vi "Create G-CLI Script VIPCApply.vi"(8 "error in (no error)":errorcluster, 10 "VIPC File Path":path, 11 "PostBuildSupport in":refnum<class "PostBuildSupport.lvclass">) -> (0 "error out":errorcluster, 2 "command":string, 3 "PostBuildSupport out":refnum<class "PostBuildSupport.lvclass">)   [LabVIEW 2019, in "PostBuildSupport.lvclass"]
uses:
  PostBuildSupport.lvclass
  PostBuildSupport.lvclass/PostBuildSupport.ctl
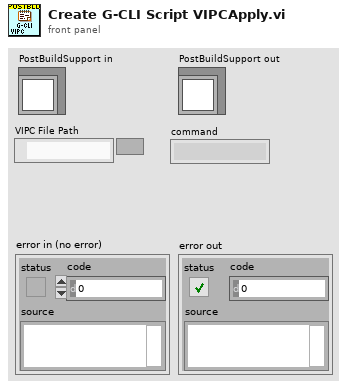
[diagram p1: front panel]
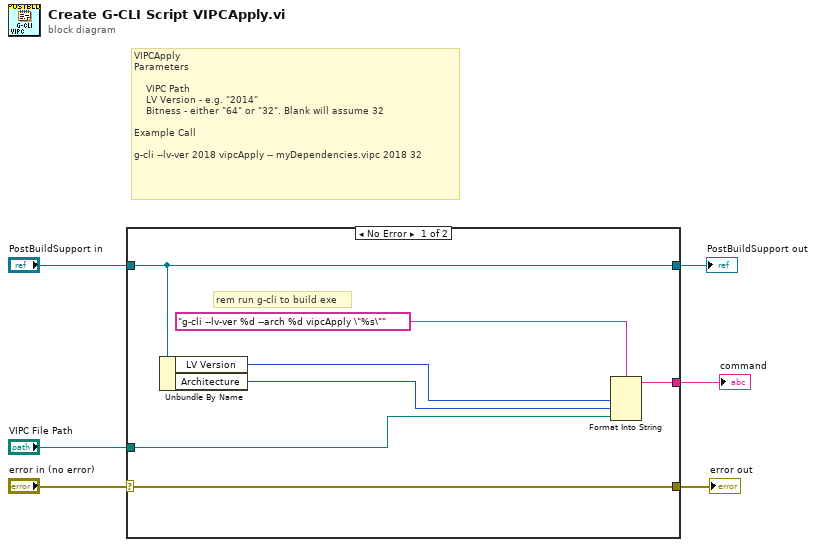
[diagram p0: block diagram]
diagram:
  # "VIPCApply\nParameters\n\n    VIPC Path\n    LV Version - e.g. \"2014\"\n    Bitness - either \"64\" or \"32\". Blank will assume 32\n\nExample Call\n\ng-cli --lv-ver 2018 vipcApply -- myDependencies.vipc 2018 32"
  n1 = case shown="No Error" "error in (no error)" {
    selector: "error in (no error)" -> [w8 w15]
    tunnel: "PostBuildSupport in" -> [w13 w14]
    tunnel: [w8 w15] -> w4
    tunnel: [w13 w14] -> w3
    tunnel: [w9 _] -> w2
    tunnel: "VIPC File Path" -> [w7 _]
    frame No Error {
      # "rem run g-cli to build exe"
      n2 = Unbundle By Name(w13) -> ("LV Version"=w11:u32, "Architecture"=w10:u32)
      n3 = Format Into String(format string="g-cli --lv-ver %d --arch %d vipcApply \"%s\"", w11, w10, w7) -> (resulting string=w9:string)  [unwired: 2 in, 1 out]
    }
    frame Error {
    }
  }
  "error out" <- w4
  "PostBuildSupport out" <- w3
  "command" <- w2
